vi "Make Default Model.vi"(8 "error in (no error)":errorcluster) -> (0 "error out":errorcluster, 3 "Result Model out":refnum<class "Result Model.lvclass">)   [LabVIEW 2020, in "Result Model Statistics.lvclass"]
uses:
  Result Model Statistics.lvclass
  source/User Interface/Result Model/Result Model.lvclass
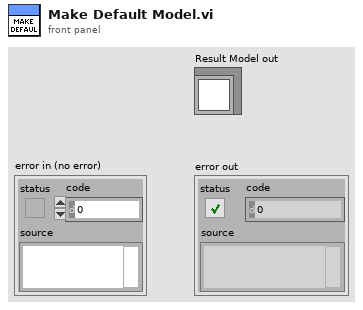
[diagram p1: front panel]
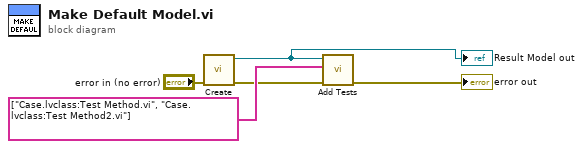
[diagram p0: block diagram]
diagram:
  n1 = call "Create.vi"("error in (no error)"="error in (no error)") -> ("error out"=w3:errorcluster, "Result Model out"=w1:refnum<class "Result Model.lvclass">)  [unwired: 9 in]
  "Result Model out" <- w1
  n2 = call "Add Tests.vi"("error in (no error)"=w3, "Tests"=string[] ["Case.lvclass:Test Method.vi", "Case.lvclass:Test Method2.vi"], "Result Model by Reference In"=w1) -> ("error out"=→"error out":errorcluster)  [unwired: 8 in]
